vi "SubVI_PostPolarisation.vi"(0 "Test References":T1, 1 "Angles":dbl[](array[numeric]), 2 "Scan Polar Params":refnum<vi>[](array[refnum])) -> ()   [LabVIEW 2019]
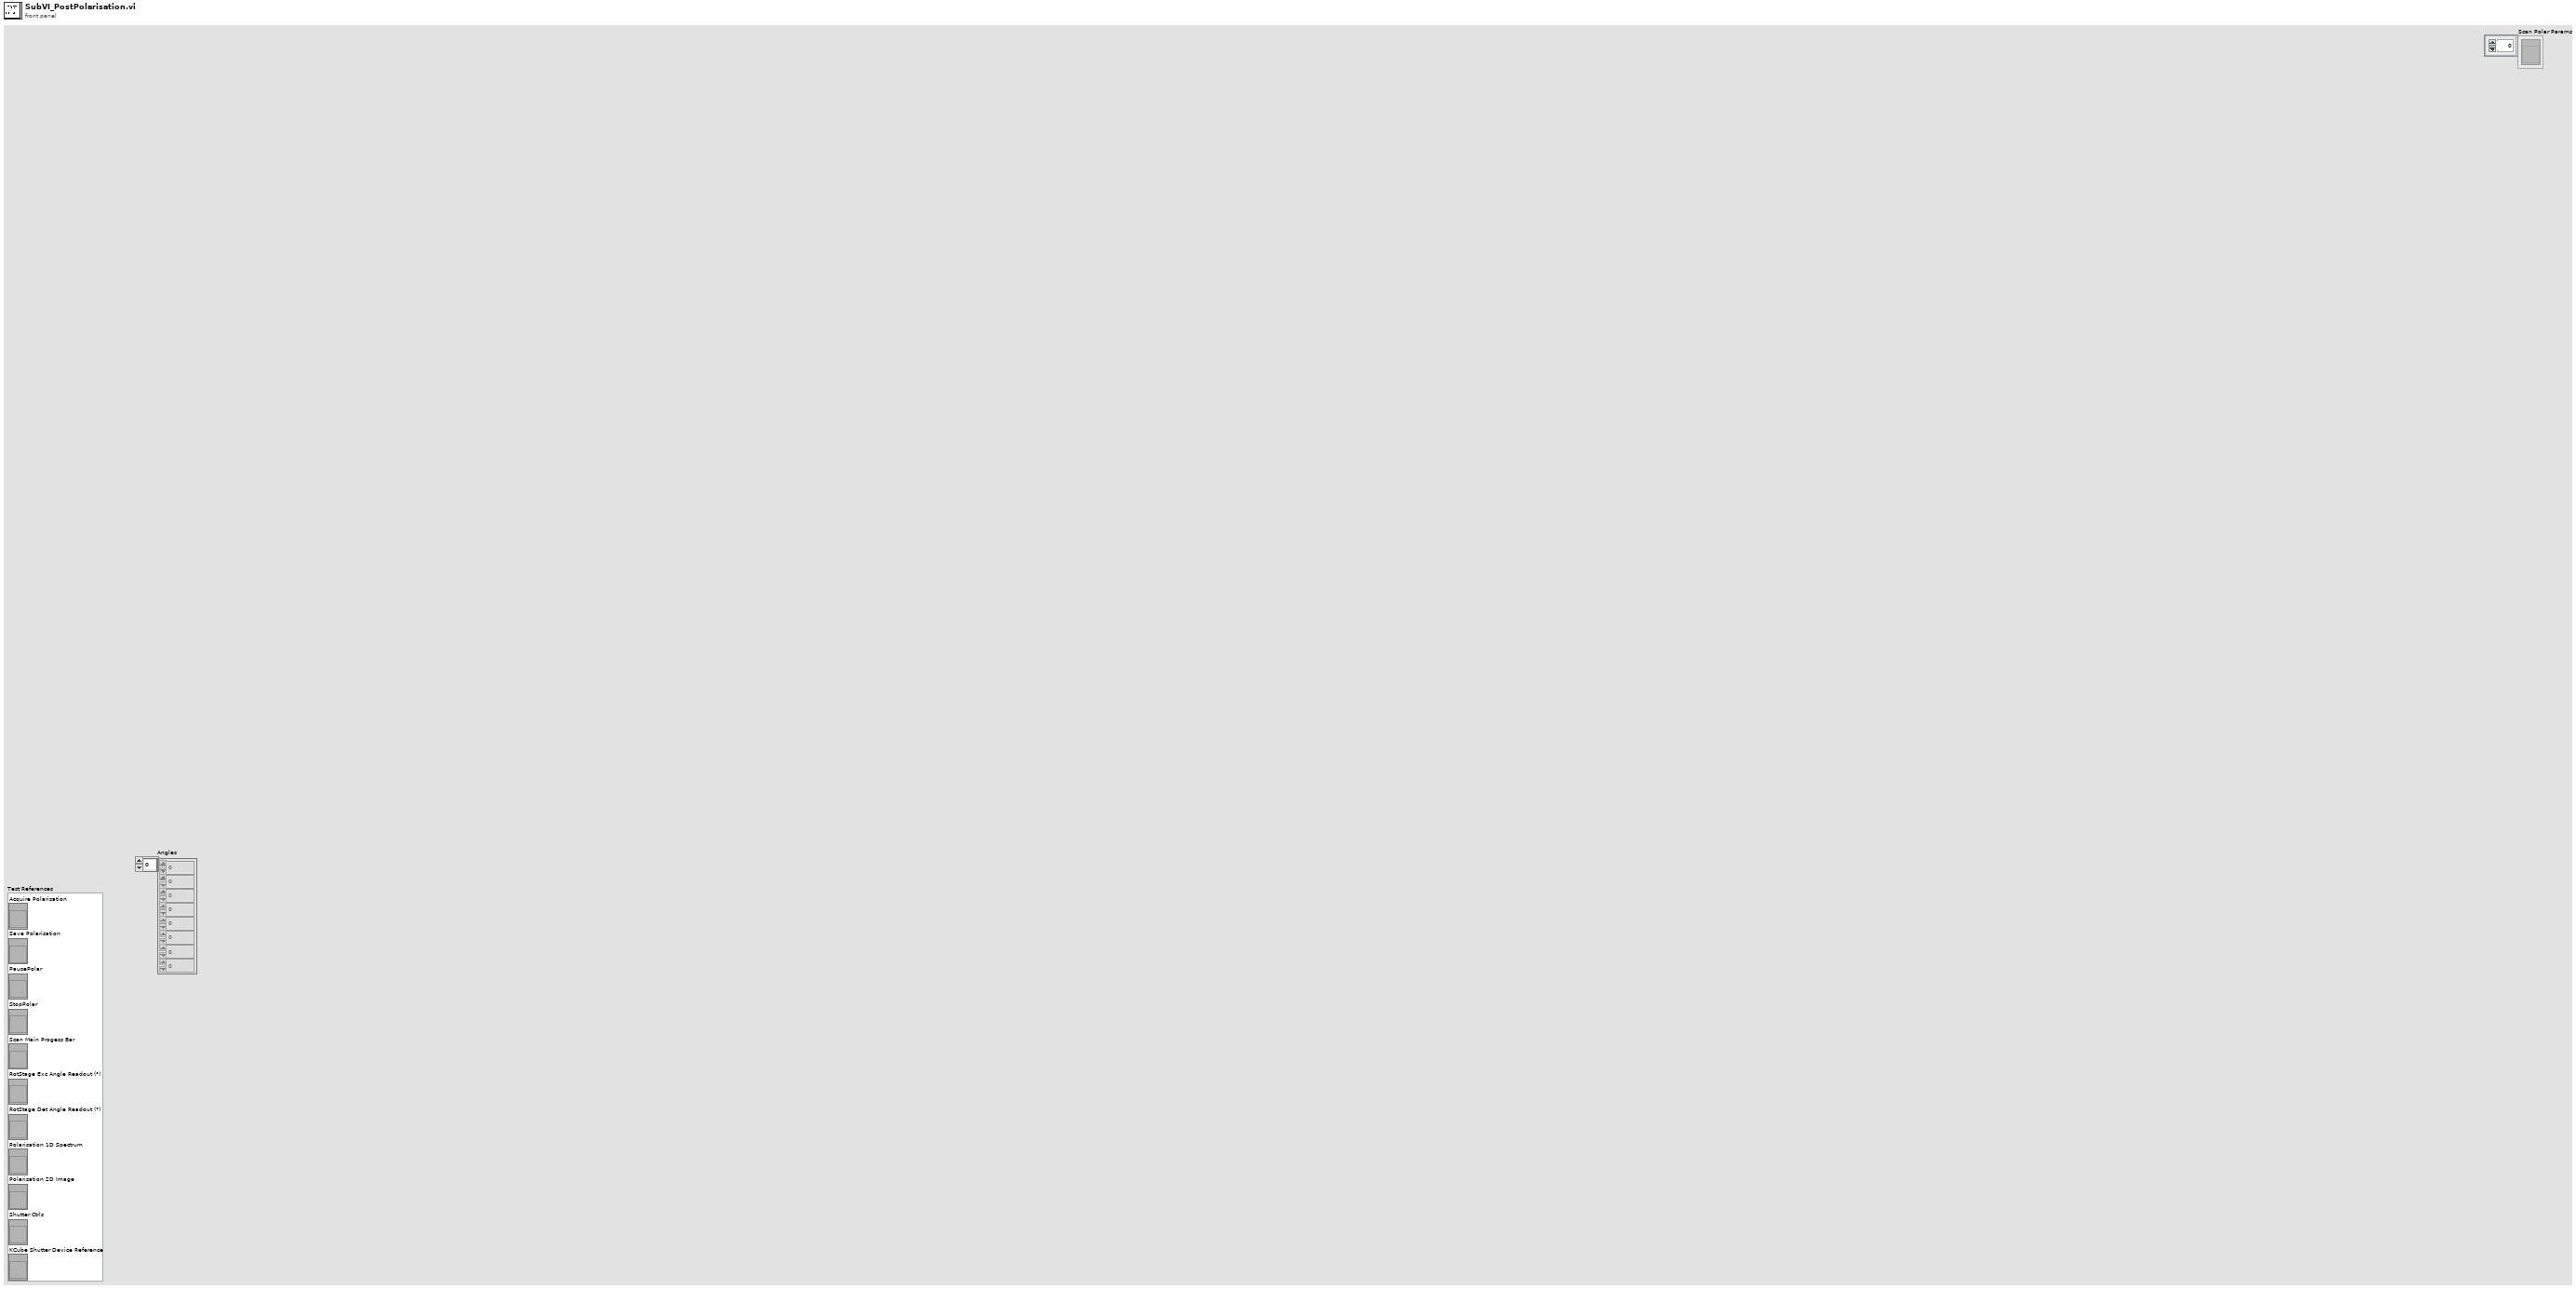
[diagram p1: front panel]
types:
  T1 = cluster{"Acquire Polarisation":refnum<vi>, "Save Polarisation":refnum<vi>, "PausePolar":refnum<vi>, "StopPolar":refnum<vi>, "Scan Main Progess Bar":refnum<vi>, "RotStage Exc Angle Readout (°)":refnum<vi>, "RotStage Det Angle Readout (°)":refnum<vi>, "Polarisation 1D Spectrum":refnum<vi>, "Polarisation 2D Image":refnum<vi>, "Shutter Ctrls":refnum<vi>, "KCube Shutter Device Reference":refnum<vi>}
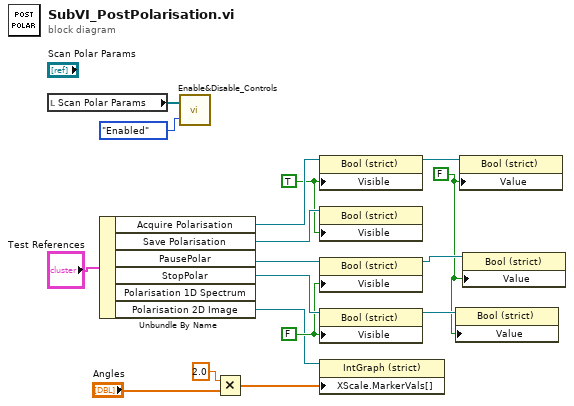
[diagram p0: block diagram]
diagram:
  w1 = FALSE ("Value")
  w11 = FALSE ("Visible")
  w12 = TRUE ("Visible")
  n1 = local read "Scan Polar Params"() -> (w10:refnum<vi>[])
  n2 = Unbundle By Name("Test References") -> ("Acquire Polarisation"=w16:refnum<vi>, "Save Polarisation"=w15:refnum<vi>, "PausePolar"=w14:refnum<vi>, "StopPolar"=w13:refnum<vi>, "Polarisation 2D Image"=w8:refnum<vi>)  [unwired: 1 out]
  n3 = call "Enable&Disable_Controls.vi"("Enum"=enum16{"Enabled", "Disabled", "Disabled&Grayed"}."Enabled", "References"=w10) -> ()  [unwired: 1 in]
  n4 = Multiply(x=2.0, y="Angles") -> (x*y=w4:dbl[])
  n5 = property class="Bool (strict)"(reference=w16, "Visible"=w12) -> (reference out=w6:refnum<vi>)  [unwired: 1 in, 1 out]
  n6 = property class="Bool (strict)"(reference=w15, "Visible"=w12) -> ()  [unwired: 1 in, 2 out]
  n7 = property class="Bool (strict)"(reference=w14, "Visible"=w11) -> (reference out=w2:refnum<vi>)  [unwired: 1 in, 1 out]
  n8 = property class="Bool (strict)"(reference=w13, "Visible"=w11) -> (reference out=w3:refnum<vi>)  [unwired: 1 in, 1 out]
  n9 = property class="IntGraph (strict)"(reference=w8, "XScale.MarkerVals[]"=w4) -> ()  [unwired: 1 in, 2 out]
  n10 = property class="Bool (strict)"(reference=w3, "Value"=w1) -> ()  [unwired: 1 in, 2 out]
  n11 = property class="Bool (strict)"(reference=w6, "Value"=w1) -> ()  [unwired: 1 in, 2 out]
  n12 = property class="Bool (strict)"(reference=w2, "Value"=w1) -> ()  [unwired: 1 in, 2 out]
